vi "基于Labview的BMI计算器.vi"() -> ()   [LabVIEW 2018]
panel:
  in  "结束运行":bool
  out "健康状况":string
  out "BMI值":dbl
  in  "输入身高/cm":dbl
  in  "输入体重/kg":dbl
  # "身体质量指数 (Body Mass Index, 简称BMI), 亦称克托莱指数, 是目前国际上常用的衡量人体胖瘦程度以及是否健康的一个标准。BMI 值超标，意味着你必须减肥了。"
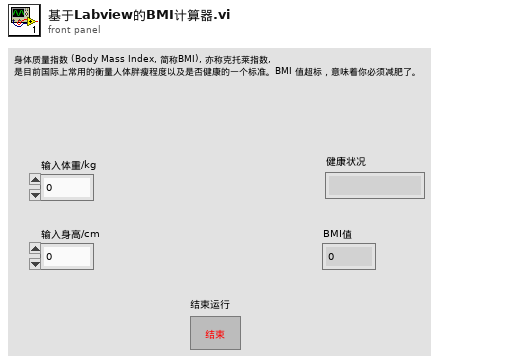
[diagram p1: front panel]
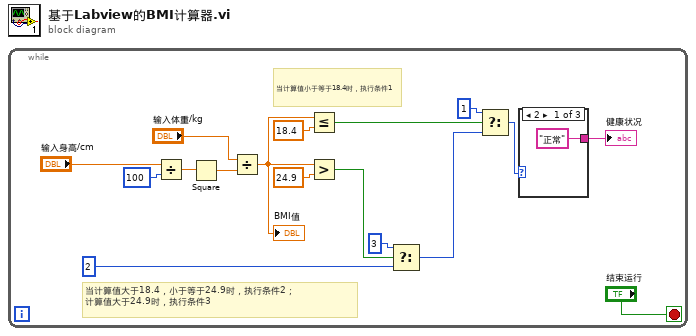
[diagram p0: block diagram]
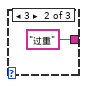
[diagram p2: hidden frame]
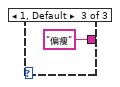
[diagram p3: hidden frame]
diagram:
  n1 = while {
    stop <- "结束运行" stop-if-true
    # "当计算值大于18.4，小于等于24.9时，执行条件2；\n计算值大于24.9时，执行条件3"
    # "当计算值小于等于18.4时，执行条件1"
    n2 = Divide(x="输入身高/cm", y=100) -> (x/y=w2:dbl)
    n3 = Square(x=w2) -> (x^2=w16:dbl)
    n4 = Divide(x="输入体重/kg", y=w16) -> (x/y=w13:dbl)
    "BMI值" <- w13
    n5 = Less Or Equal?(x=w13, y=18.4) -> (x <= y?=w11:bool)
    n6 = Greater?(x=w13, y=24.9) -> (0:w9:bool)
    n7 = Select(t=3, s=w9, f=2) -> (s? t:f=w10:i32)
    n8 = Select(t=1, s=w11, f=w10) -> (s? t:f=w6:i32)
    n9 = case shown="2" w6 {
      tunnel: ["正常" "过重" "偏瘦"] -> w5
      frame 2 {
      }
      frame 3 {
      }
      frame 1, Default {
      }
    }
    "健康状况" <- w5
  }
